vi "MoveV.vi"() -> ()   [LabVIEW 2019]
uses:
  <vilib>/addons/control/pid/pid.llb/PID (DBL).vi
  <vilib>/addons/control/pid/NI_PID_pid.lvlib
panel:
  in  "OBJ":dbl[](array[numeric])
  in  "PID gains":T1={"proportional gain (Kc)"=0.6, "integral time (Ti, min)"=0.0, "derivative time (Td, min)"=0.0002}
  in  "output range":cluster{"output high":dbl, "output low":dbl}={"output high"=100.0, "output low"=-100.0}
  in  "EncRst":bool
  out "差值":dbl[](array[numeric])
  out "Enc":dbl[](array[numeric])
  in  "dt (s)":dbl=0.010000000000000002 format="%#_13g"
  in  "reinitialize? (F)":bool
  out "power":dbl[](array[numeric])
  in  "stop":bool
  out "error out":errorcluster
  in  "error in (no error)":errorcluster
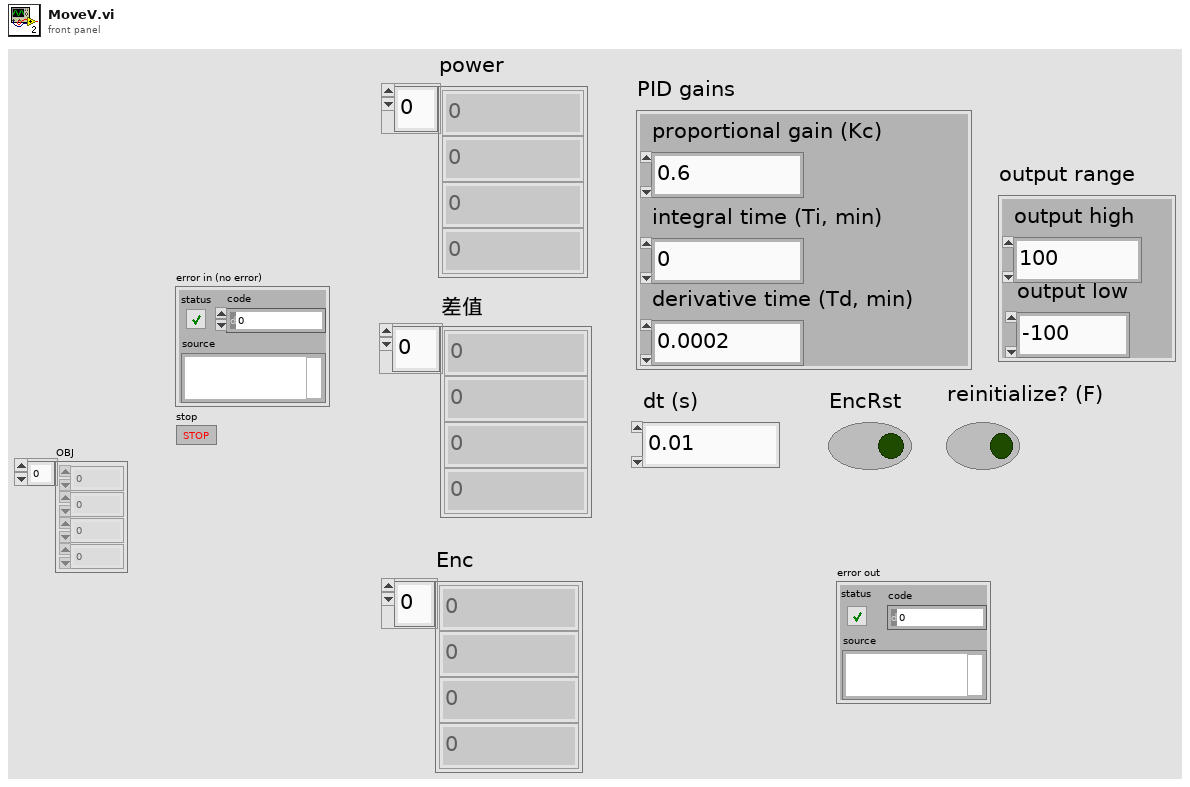
[diagram p1: front panel]
types:
  T1 = cluster{"proportional gain (Kc)":dbl, "integral time (Ti, min)":dbl, "derivative time (Td, min)":dbl}
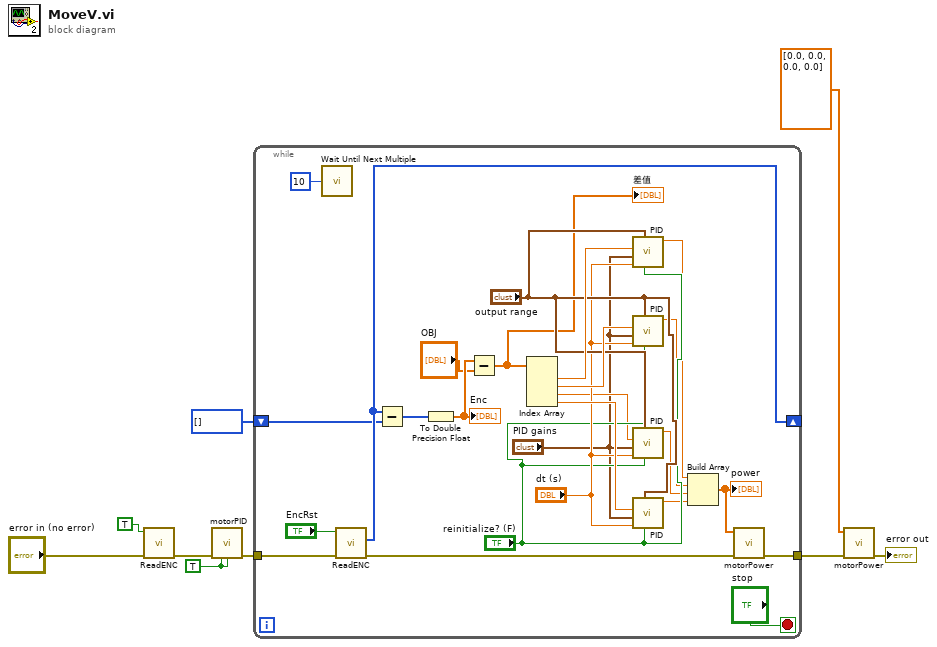
[diagram p0: block diagram]
diagram:
  w9 = TRUE ("EncRst")
  n1 = call "ReadENC.vi"("error in (no error)"="error in (no error)", "Reset"=TRUE) -> ("error out"=w8:errorcluster)  [unwired: 8 in, 1 out]
  n2 = call "motorPID.vi"("error in (no error)"=w8, "reinitialize? (F)"=w9, "EncRst"=w9) -> ("error out"=w3:errorcluster)  [unwired: 9 in, 3 out]
  n3 = while {
    tunnel: w3 -> [w17]
    tunnel: [w16] -> w4
    shift-right: [w11] -> _
    shift-left: i32[] [] ("ENC") -> [w10]
    stop <- "stop" stop-if-true
    n4 = call "Wait Until Next Multiple"("Count(mSec)"=u32 10) -> ()  [unwired: 1 out]
    n5 = call "ReadENC.vi"("error in (no error)"=w17, "Reset"="EncRst") -> ("error out"=w29:errorcluster, "ENC"=w11:i32[])  [unwired: 8 in]
    n6 = Subtract(x=w11, y=w10) -> (x-y=w15:i32[])
    n7 = To Double Precision Float(number=w15) -> (double precision float=w13:dbl[])
    "Enc" <- w13
    n8 = Subtract(x=w13, y="OBJ") -> (x-y=w14:dbl[])
    "差值" <- w14
    n9 = Index Array(array=w14) -> (element #1=w32:dbl, element #2=w31:dbl, element #3=w23:dbl, element #4=w26:dbl)  [unwired: 4 in]
    n10 = call-poly <vilib>:"PID.vi"("reinitialize? (F)"="reinitialize? (F)", "output range"="output range", "dt (s)"="dt (s)", "PID gains"="PID gains", "process variable"=w32) -> ("output"=w20:dbl)  [unwired: 5 in, 1 out]
    n11 = call-poly <vilib>:"PID.vi"("reinitialize? (F)"="reinitialize? (F)", "output range"="output range", "dt (s)"="dt (s)", "PID gains"="PID gains", "process variable"=w31) -> ("output"=w21:dbl)  [unwired: 5 in, 1 out]
    n12 = call-poly <vilib>:"PID.vi"("reinitialize? (F)"="reinitialize? (F)", "output range"="output range", "dt (s)"="dt (s)", "PID gains"="PID gains", "process variable"=w23) -> ("output"=w19:dbl)  [unwired: 5 in, 1 out]
    n13 = call-poly <vilib>:"PID.vi"("reinitialize? (F)"="reinitialize? (F)", "output range"="output range", "dt (s)"="dt (s)", "PID gains"="PID gains", "process variable"=w26) -> ("output"=w18:dbl)  [unwired: 5 in, 1 out]
    n14 = Build Array(w20, w21, w19, w18) -> (w28:dbl[])
    "power" <- w28
    n15 = call "motorPower.vi"("error in (no error)"=w29, "DC_Pwr"=w28) -> ("error out"=w16:errorcluster)  [unwired: 9 in]
  }
  n16 = call "motorPower.vi"("error in (no error)"=w4, "DC_Pwr"=dbl[] [0.0, 0.0, 0.0, 0.0]) -> ("error out"=→"error out":errorcluster)  [unwired: 9 in]
